vi "Check If Custom Device Enabled.vi"(8 "error in":errorcluster, 11 "Ballard MIL-STD 1553 custom device in":T1 format="%.0x") -> (0 "error out":errorcluster, 2 "Is Custom Device Enabled?":bool, 3 "Ballard MIL-STD 1553 custom device out":T1 format="%.0x")   [LabVIEW 2020, in "Ballard MIL-STD-1553 Scripting.lvlib"]
uses:
  Ballard MIL-STD-1553 Scripting.lvlib
  <vilib>/NI VeriStand/Custom Device API/Custom Device API.lvlib
  Constants.vi
  <vilib>/NI VeriStand/Custom Device API/Custom Device Item Ref.ctl
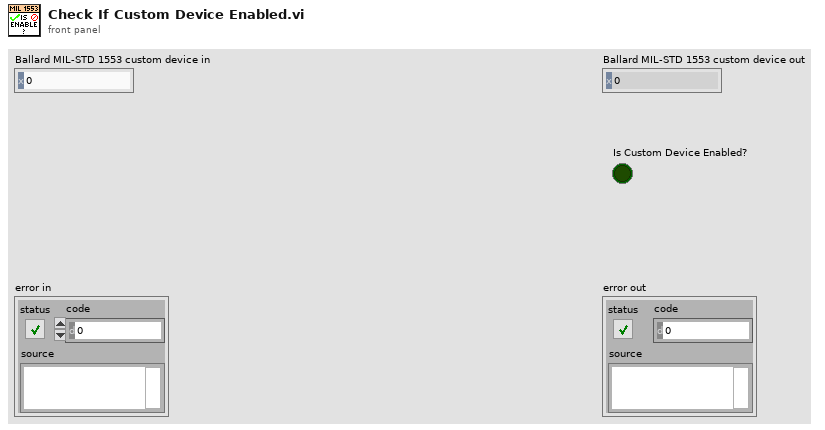
[diagram p1: front panel]
types:
  T1 = typedef "Custom Device API.lvlib/Custom Device Item Ref.ctl" = u64
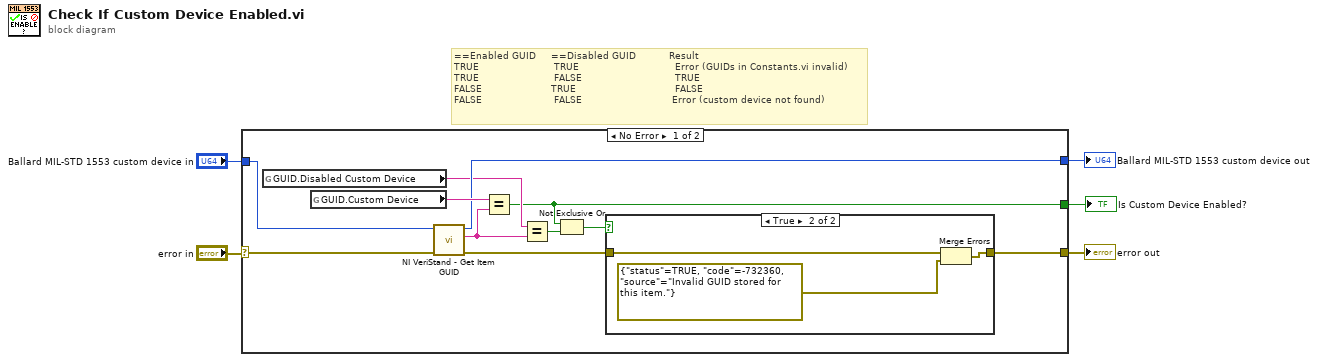
[diagram p0: block diagram]
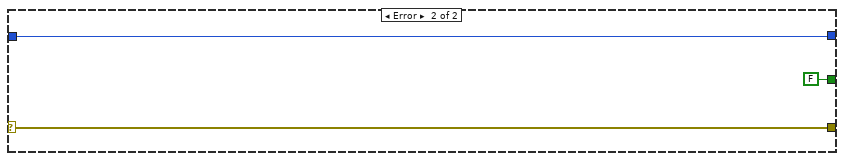
[diagram p3: hidden frame]
diagram:
  # "==Enabled GUID     ==Disabled GUID           Result\nTRUE                         TRUE                                Error (GUIDs in Constants.vi invalid)\nTRUE                         FALSE                               TRUE\nFALSE                       TRUE                                 FALSE\nFALSE                        FALSE                              Error (custom device not found)"
  n1 = case shown="No Error" "error in" {
    selector: "error in" -> [w16 w22]
    tunnel: [w13 w23] -> w4
    tunnel: "Ballard MIL-STD 1553 custom device in" -> [w12 w23]
    tunnel: [w8 FALSE] -> w2
    tunnel: [w6 w22] -> w1
    frame No Error {
      n2 = global read "Constants.vi" "GUID.Disabled Custom Device"() -> (w11:string)
      n3 = global read "Constants.vi" "GUID.Custom Device"() -> (w14:string)
      n4 = call <vilib>:"NI VeriStand - Get Item GUID.vi"("error in (no error)"=w16, "Item Ref in"=w12) -> ("error out"=w15:errorcluster, "GUID"=w10:string, "Item Ref out"=w13:T1)  [unwired: 7 in]
      n5 = Equal?(x=w14, y=w10) -> (x = y?=w8:bool)
      n6 = Equal?(x=w11, y=w10) -> (x = y?=w9:bool)
      n7 = Not Exclusive Or(1:w9, 2:w8) -> (0:w7:bool)
      n8 = case shown="True" w7 {
        tunnel: [w17 w19] -> w6
        tunnel: w15 -> [w17 w18]
        frame False {
        }
        frame True {
          n9 = Merge Errors(w18, errorcluster {"status"=TRUE, "code"=-732360, "source"="Invalid GUID stored for this item."} ("New Error")) -> (w19:errorcluster)
        }
      }
    }
    frame Error {
    }
  }
  "Ballard MIL-STD 1553 custom device out" <- w4
  "error out" <- w1
  "Is Custom Device Enabled?" <- w2
